vi "InitiateQueues.vi"() -> (1 "Queue References":T1)   [LabVIEW 2013]
doc: "Initializes all the queues that will be used to pass data, mostly objective-related, around.\n\nElizabeth Mahon and team, 4/12/2014"
uses:
  Data/TypeDefs/Queues.ctl
  Logic/Classes/Waypoint/Waypoint.lvclass
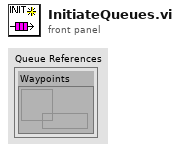
[diagram p1: front panel]
types:
  T1 = typedef "Queues.ctl" = cluster{"Waypoints":refnum<queue>}
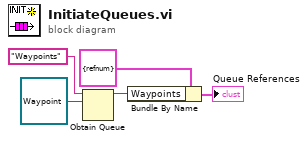
[diagram p0: block diagram]
diagram:
  n1 = Obtain Queue(name (unnamed)="Waypoints", element data type=refnum<class "Waypoint.lvclass"> refnum ("Waypoint.lvclass")) -> (queue out=w3:refnum<queue>)  [unwired: 3 in, 2 out]
  n2 = Bundle By Name(cluster=T1 {"Waypoints"=refnum} ("input cluster"), "Waypoints"=w3) -> (→"Queue References":T1)
